vi "m_open.vi"(2 "error in (no error)":errorcluster, 3 "configuration file path":path) -> (0 "error out":errorcluster, 1 "configuration file path copy":path)   [LabVIEW 2017]
doc: "Write Cornerstone persitant data to configuration (INI) file."
uses:
  m_globals.vi
  <vilib>/Utility/config.llb/NI_LVConfig.lvlib
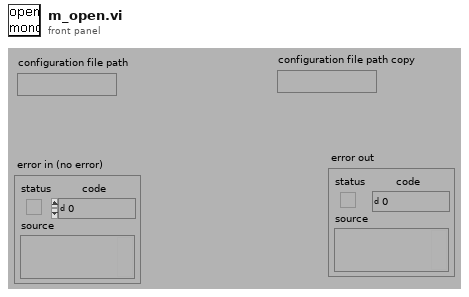
[diagram p1: front panel]
types:
  T1 = typedef "NI_LVConfig.lvlib/Config Data RefNum.ctl" = refnum<k1>
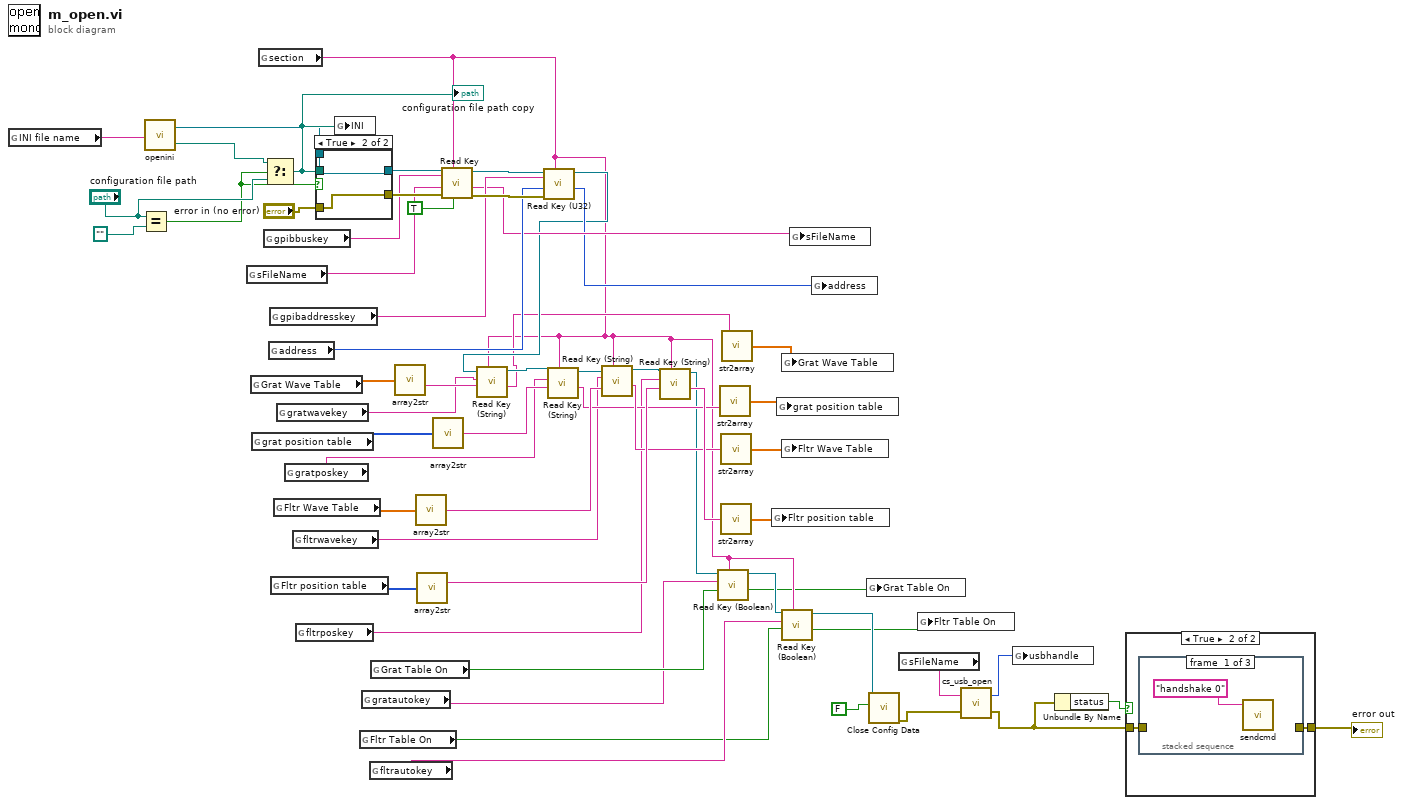
[diagram p0: block diagram]
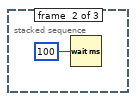
[diagram p3: hidden frame]
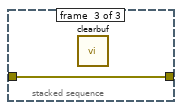
[diagram p4: hidden frame]
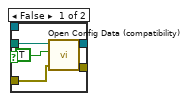
[diagram p5: hidden frame]
diagram:
  n1 = global read "m_globals.vi" "INI file name"() -> (w11:string)
  n2 = Equal?(x="configuration file path", y=path "") -> (x = y?=w9:bool)
  n3 = call "openini.vi"("INI file name"=w11) -> ("refnum"=w8:refnum<k1>, "appended path"=w10:path)
  n4 = global read "m_globals.vi" "sFileName"() -> (w53:string)
  n5 = global read "m_globals.vi" "Grat Wave Table"() -> (w44:dbl[])
  n6 = global read "m_globals.vi" "grat position table"() -> (w43:u16[])
  n7 = global read "m_globals.vi" "section"() -> (w20:string)
  n8 = global read "m_globals.vi" "gpibbuskey"() -> (w54:string)
  n9 = Select(t=w10, s=w9, f="configuration file path") -> (s? t:f=w12:path)
  "configuration file path copy" <- w12
  n10 = global read "m_globals.vi" "address"() -> (w51:i16)
  n11 = global read "m_globals.vi" "gpibaddresskey"() -> (w52:string)
  n12 = global read "m_globals.vi" "Fltr position table"() -> (w37:u16[])
  n13 = global read "m_globals.vi" "Fltr Wave Table"() -> (w38:dbl[])
  n14 = global read "m_globals.vi" "gratwavekey"() -> (w28:string)
  n15 = global read "m_globals.vi" "gratposkey"() -> (w27:string)
  n16 = global read "m_globals.vi" "fltrwavekey"() -> (w26:string)
  n17 = global read "m_globals.vi" "fltrposkey"() -> (w25:string)
  n18 = case shown="True" w9 {
    tunnel: [w65 w66] -> w60
    tunnel: "error in (no error)" -> [w64 w67]
    tunnel: [w63 w67] -> w58
    tunnel: w12 -> [w61 _]
    tunnel: w8 -> [_ w66]
    frame False {
      n19 = call <vilib>:"Open Config Data (compatibility).vi"("error in (no error)"=w64, "create file if necessary (T)"=TRUE ("create file if necessary? (T)"), "configuration file path"=w61) -> ("error out"=w63:errorcluster, "refnum"=w65:T1)  [unwired: 6 in, 1 out]
    }
    frame True {
    }
  }
  n20 = global write "m_globals.vi" "INI"(w12) -> ()
  n21 = global read "m_globals.vi" "Fltr Table On"() -> (w15:bool)
  n22 = global read "m_globals.vi" "gratautokey"() -> (w22:string)
  n23 = global read "m_globals.vi" "fltrautokey"() -> (w16:string)
  n24 = global read "m_globals.vi" "Grat Table On"() -> (w23:bool)
  n25 = call "array2str.vi"("array in"=w44) -> ("string out"=w41:string)
  n26 = call "array2str.vi"("array in"=w38) -> ("string out"=w35:string)
  n27 = call "array2str.vi"("array in"=w37) -> ("string out"=w34:string)
  n28 = call "array2str.vi"("array in"=w43) -> ("string out"=w39:string)
  n29 = call-poly <vilib>:"Read Key.vi"("read raw string? (F)"=TRUE, "section"=w20, "error in (no error)"=w58, "default value"=w53, "key"=w54, "refnum"=w60) -> ("error out"=w57:errorcluster, "value"=w50:string, "refnum out"=w56:T1)  [unwired: 2 in, 1 out]
  n30 = call <vilib>:"Read Key (U32).vi"("section"=w20, "error in (no error)"=w57, "default value"=w51, "key"=w52, "refnum"=w56) -> ("value"=w49:u32, "refnum out"=w42:T1)  [unwired: 3 in, 2 out]
  n31 = call <vilib>:"Read Key (String).vi"("section"=w20, "default value"=w41, "key"=w28, "refnum"=w42) -> ("value"=w30:string, "refnum out"=w40:T1)  [unwired: 4 in, 2 out]
  n32 = call <vilib>:"Read Key (String).vi"("section"=w20, "default value"=w39, "key"=w27, "refnum"=w40) -> ("value"=w29:string, "refnum out"=w36:T1)  [unwired: 4 in, 2 out]
  n33 = call <vilib>:"Read Key (String).vi"("section"=w20, "default value"=w35, "key"=w26, "refnum"=w36) -> ("value"=w32:string, "refnum out"=w31:T1)  [unwired: 4 in, 2 out]
  n34 = call <vilib>:"Read Key (String).vi"("section"=w20, "default value"=w34, "key"=w25, "refnum"=w31) -> ("value"=w33:string, "refnum out"=w24:T1)  [unwired: 4 in, 2 out]
  n35 = call <vilib>:"Read Key (Boolean).vi"("section"=w20, "default value"=w23, "key"=w22, "refnum"=w24) -> ("value"=w17:bool, "refnum out"=w21:T1)  [unwired: 4 in, 2 out]
  n36 = call "str2array.vi"("string in"=w29) -> ("array out"=w47:dbl[])
  n37 = call "str2array.vi"("string in"=w32) -> ("array out"=w46:dbl[])
  n38 = call "str2array.vi"("string in"=w33) -> ("array out"=w45:dbl[])
  n39 = call "str2array.vi"("string in"=w30) -> ("array out"=w48:dbl[])
  n40 = global write "m_globals.vi" "Fltr position table"(w45) -> ()
  n41 = global write "m_globals.vi" "grat position table"(w47) -> ()
  n42 = global write "m_globals.vi" "Grat Wave Table"(w48) -> ()
  n43 = global write "m_globals.vi" "Fltr Wave Table"(w46) -> ()
  n44 = call <vilib>:"Read Key (Boolean).vi"("section"=w20, "default value"=w15, "key"=w16, "refnum"=w21) -> ("value"=w18:bool, "refnum out"=w19:T1)  [unwired: 4 in, 2 out]
  n45 = global write "m_globals.vi" "sFileName"(w50) -> ()
  n46 = global write "m_globals.vi" "address"(w49) -> ()
  n47 = global write "m_globals.vi" "Grat Table On"(w17) -> ()
  n48 = call <vilib>:"Close Config Data.vi"("write file if changed (T)"=FALSE ("write configuration file? (F)"), "refnum"=w19) -> ("error out"=w7:errorcluster)  [unwired: 8 in, 1 out]
  n49 = global read "m_globals.vi" "sFileName"() -> (w6:string)
  n50 = global write "m_globals.vi" "Fltr Table On"(w18) -> ()
  n51 = call "cs_usb_open.vi"("error in"=w7, "sFileName"=w6) -> ("error out"=w2:errorcluster, "handle"=w5:i32)
  n52 = global write "m_globals.vi" "usbhandle"(w5) -> ()
  n53 = Unbundle By Name(w2) -> ("status"=w4:bool)
  n54 = case shown="True" w4 {
    tunnel: w2 -> [w68 w70]
    tunnel: [w68 w69] -> w3
    frame False {
    }
    frame True {
      n55 = stacked-sequence {
        tunnel: w70 -> [_ _ w73]
        tunnel: [_ _ w73] -> w69
        frame #0 {
          n56 = call "sendcmd.vi"("command in"="handshake 0") -> ()  [unwired: 2 in, 1 out]
        }
        frame #1 {
          n57 = Wait (ms)(milliseconds to wait=u32 100) -> ()  [unwired: 1 out]
        }
        frame #2 {
          n58 = call "clearbuf.vi"() -> ()  [unwired: 1 in, 1 out]
        }
      }
    }
  }
  "error out" <- w3
